vi "SPD.Strobe Phase setup.vi"(5 "Graph":refnum<vi>, 7 "Progress":refnum<vi>, 8 "Error In":errorcluster, 11 "SPD.Stand Ctrl in":T1 {"spdDeviceSession"."hidSPD.Controller"."HV_bias" format="%#_6p, V"; "spdDeviceSession"."hidSPD.Controller"."TSet" format="%#_6p, DegC"}) -> (0 "Error Out":errorcluster, 1 "pass":bool, 2 "result":string, 3 "SPD.Stand Ctrl out":T1 {"spdDeviceSession"."hidSPD.Controller"."HV_bias" format="%#_6p, V"; "spdDeviceSession"."hidSPD.Controller"."TSet" format="%#_6p, DegC"})   [LabVIEW 2018]
uses:
  typedefs/SPD.Stand Ctrl.ctl
  Instruments/SPD HID Interface/hidSPDLibForLabView/LibVIs/hidSPD Controls/hidSPD Device Session.ctl
  Instruments/SPD HID Interface/hidSPDLibForLabView/LibVIs/hidSPD Controls/hidSPD Controller.ctl
  Instruments/KC705 DevBoard/typedefs/DevB.Session.ctl
  Instruments/KeySight 53230A/typedefs/FreqC.Session.ctl
  Instruments/KeySight 8164B/KeySight 8164B LAN InstrLib/typedefs/KeySight 8164B control.ctl
  Instruments/LeCroy SDA830/typedefs/LeCroy.Session.ctl
  typedefs/SPD.Events.ctl
  Instruments/KeySight 8164B/KeySight 8164B LAN InstrLib/typedefs/KeySight 8164B Power Unit.ctl
  <vilib>/Utility/error.llb/Error Cluster From Error Code.vi
  <vilib>/ErrorRing/Error Ring.xnode
  Instruments/KeySight 8164B/KeySight 8164B LAN InstrLib.lvlib
  Instruments/SPD HID Interface/hidSPDLibForLabView/hidSPDLibForLabView.lvlib
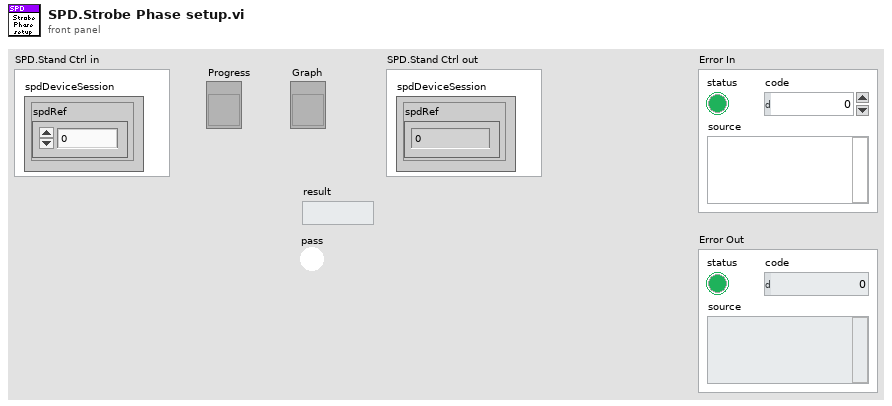
[diagram p1: front panel]
types:
  T1 = typedef "SPD.Stand Ctrl.ctl" = cluster{"spdDeviceSession":T2, "DevBSession":T4, "FreqCSession":T5, "8164BSession":T6, "LeCroySession":T7, "Events":T8}
  T2 = typedef "hidSPDLibForLabView.lvlib/hidSPD Device Session.ctl" = cluster{"spdRef":u64, "connected":bool, "spdName":string, "hidSPD.Controller":T3}
  T3 = typedef "hidSPDLibForLabView.lvlib/hidSPD Controller.ctl" = cluster{"TSet":sgl, "HV_bias":sgl, "DDS_stb_code":u16}
  T4 = typedef "DevB.Session.ctl" = cluster{"DevBRef":refnum<visa-resource-name>, "connected":bool}
  T5 = typedef "FreqC.Session.ctl" = cluster{"FreqCRef":refnum<visa-resource-name>, "timeout":dbl, "connected":bool}
  T6 = typedef "KeySight 8164B LAN InstrLib.lvlib/KeySight 8164B control.ctl" = cluster{"Connection ID":refnum<k5>, "Connected":bool, "Info":string, "Slots Info":string[]}
  T7 = typedef "LeCroy.Session.ctl" = cluster{"LeCroySession":refnum<visa-resource-name>, "connected":bool}
  T8 = typedef "SPD.Events.ctl" = cluster{"DCRTest":refnum<user-event>, "Stop":refnum<user-event>}
  T9 = typedef "KeySight 8164B LAN InstrLib.lvlib/KeySight 8164B Power Unit.ctl" = enum16{"dBm", "Watt"}
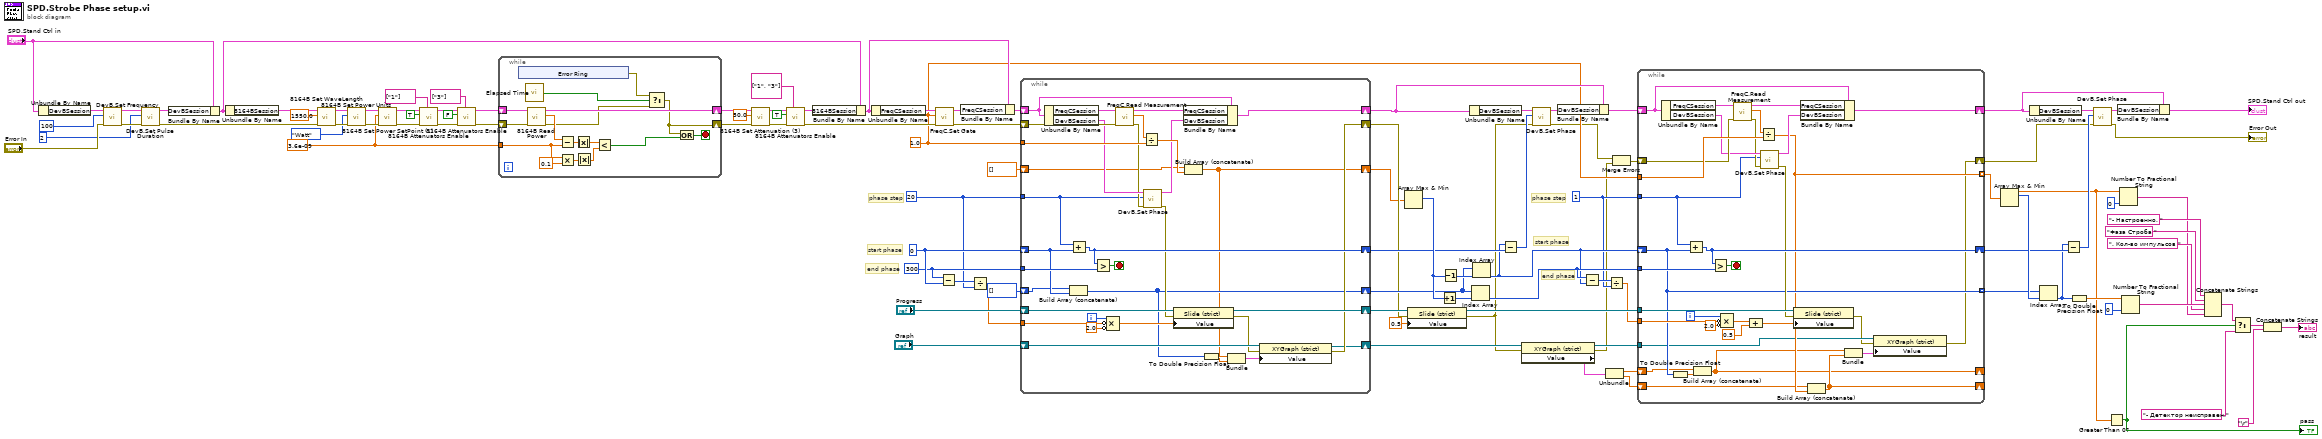
[diagram p0: block diagram]
diagram:
  w15 = 1 ("delta")
  w77 = 3.6e-09 ("Power")
  w45 = 1.0 ("Gate, sec")
  w25 = 20 ("delta")
  w27 = 300 ("HV_bias")
  w28 = 0 ("HV_bias")
  # "end phase"
  # "start phase"
  # "phase step"
  # "end phase"
  # "start phase"
  # "phase step"
  n1 = Unbundle By Name("SPD.Stand Ctrl in") -> ("DevBSession"=w94:T4)
  n2 = call "DevB.Set Frequency.vi"("error in (no error)"="Error In", "Frequency"=100, "DevB Session in"=w94) -> ("error out"=w90:errorcluster, "DevB Session out"=w91:T4)  [unwired: 7 in]
  n3 = call "DevB.Set Pulse Duration.vi"("error in (no error)"=w90, "Pulse Duration"=2, "DevB Session in"=w91) -> ("error out"=w78:errorcluster, "DevB Session out"=w69:T4)  [unwired: 7 in]
  n4 = Bundle By Name(cluster="SPD.Stand Ctrl in", "DevBSession"=w69) -> (w68:T1)
  n5 = Unbundle By Name(w68) -> ("8164BSession"=w67:T6)
  n6 = call "8164B Set WaveLength.vi"("error in"=w78, "WaveLength, nm"=1550.0, "KeySight 8164B control in"=w67) -> ("error out"=w86:errorcluster, "KeySight 8164B control out"=w87:T6)  [unwired: 7 in]
  n7 = call "8164B Set Power Units.vi"("error in"=w86, "Power Unit"=KeySight_8164B_Power_Unit."Watt", "KeySight 8164B control in"=w87) -> ("error out"=w84:errorcluster, "KeySight 8164B control out"=w85:T6)  [unwired: 7 in]
  n8 = call "8164B Set Power SetPoint (1).vi"("error in"=w84, "Power Set Point"=w77, "KeySight 8164B control in"=w85) -> ("error out"=w82:errorcluster, "KeySight 8164B control out"=w83:T6)  [unwired: 7 in]
  n9 = call "8164B Attenuators Enable.vi"("Slots"=string[] ["1"], "error in"=w82, "Enable"=TRUE, "KeySight 8164B control in"=w83) -> ("error out"=w58:errorcluster, "KeySight 8164B control out"=w60:T6)  [unwired: 6 in]
  n10 = call "8164B Attenuators Enable.vi"("Slots"=string[] ["3"], "error in"=w58, "Enable"=FALSE, "KeySight 8164B control in"=w60) -> ("error out"=w57:errorcluster, "KeySight 8164B control out"=w59:T6)  [unwired: 6 in]
  n11 = while {
    shift-right: [w122] -> w75
    shift-left: w59 -> [w124]
    shift-right: [w111] -> w74
    shift-left: w57 -> [w123]
    tunnel: w77 -> [w115]
    stop <- w113 stop-if-true
    n12 = xnode "Error Ring"() -> ("error out"=w109:errorcluster)
    n13 = call "Elapsed Time"() -> ("Time has Elapsed"=w110:bool)  [unwired: 12 in, 7 out]
    n14 = call "8164B Read Power.vi"("error in"=w123, "KeySight 8164B control in"=w124) -> ("error out"=w112:errorcluster, "Power"=w116:dbl, "KeySight 8164B control out"=w122:T6)  [unwired: 7 in]
    n15 = Subtract(x=w116, y=w115) -> (x-y=w121:dbl)
    n16 = Multiply(x=w115, y=0.1) -> (x*y=w119:dbl)
    n17 = Absolute Value(x=w121) -> (abs(x)=w118:dbl)
    n18 = Absolute Value(x=w119) -> (abs(x)=w117:dbl)
    n19 = Less?(x=w118, y=w117) -> (x < y?=w114:bool)
    n20 = Select(t=w109, s=w110, f=w112) -> (s? t:f=w111:errorcluster)
    n21 = Compound Arithmetic op=OR(w111, w114) -> (w113:bool)
  }
  n22 = call "8164B Set Attenuation (3).vi"("error in"=w74, "Att 3, dB"=50.0, "KeySight 8164B control in"=w75) -> ("error out"=w72:errorcluster, "KeySight 8164B control out"=w73:T6)  [unwired: 7 in]
  n23 = call "8164B Attenuators Enable.vi"("Slots"=string[] ["1", "3"], "error in"=w72, "Enable"=TRUE, "KeySight 8164B control in"=w73) -> ("error out"=w64:errorcluster, "KeySight 8164B control out"=w66:T6)  [unwired: 6 in]
  n24 = Bundle By Name(cluster=w68, "8164BSession"=w66) -> (w63:T1)
  n25 = Unbundle By Name(w63) -> ("FreqCSession"=w65:T5)
  n26 = call "FreqC.Set Gate.vi"("error In"=w64, "Gate, sec"=w45, "FreqC Session in"=w65) -> ("error out"=w102:errorcluster, "FreqC Session out"=w62:T5)  [unwired: 7 in]
  n27 = Subtract(x=w27, y=w28) -> (x-y=w26:i32)
  n28 = Bundle By Name(cluster=w63, "FreqCSession"=w62) -> (w61:T1)
  n29 = Divide(x=w26, y=w25) -> (x/y=w23:dbl)
  n30 = while {
    shift-right: [w136] -> w21
    shift-left: w102 -> [w157]
    shift-right: [w162] -> w48
    shift-left: w61 -> [w156]
    tunnel: w45 -> [w159]
    tunnel: w25 -> [w147]
    shift-right: [w149] -> w51
    shift-left: w28 -> [w148]
    tunnel: w27 -> [w151]
    shift-right: [w144] -> w22
    shift-left: "Progress" -> [w146]
    tunnel: w23 -> [w142]
    shift-right: [w130] -> w8
    shift-left: dbl[] [] -> [w139]
    shift-right: [w135] -> w10
    shift-left: "Graph" -> [w138]
    shift-right: [w131] -> w35
    shift-left: i32[] [] ("HV_bias") -> [w133]
    i -> [w143]
    stop <- w150 stop-if-true
    n31 = Unbundle By Name(w156) -> ("FreqCSession"=w161:T5, "DevBSession"=w153:T4)
    n32 = Build Array (concatenate)(w133, w148) -> (w131:i32[])
    n33 = Add(x=w147, y=w148) -> (x+y=w149:i32)
    n34 = Greater?(x=w149, y=w151) -> (0:w150:bool)
    n35 = Compound Arithmetic op=MULTIPLY(w143, invert w142, invert 2.0 ("value")) -> (w140:dbl)
    n36 = call "FreqC.Read Measurement.vi"("error In"=w157, "FreqC Session in"=w161) -> ("error out"=w152:errorcluster, "Measurement"=w160:dbl, "FreqC Session out"=w155:T5)  [unwired: 7 in]
    n37 = Divide(x=w160, y=w159) -> (x/y=w158:dbl)
    n38 = call "DevB.Set Phase.vi"("error in (no error)"=w152, "Phase"=w147, "DevB Session in"=w153) -> ("error out"=w145:errorcluster, "DevB Session out"=w154:T4)  [unwired: 7 in]
    n39 = property class="Slide (strict)"(reference=w146, error in=w145, "Value"=w140) -> (reference out=w144:refnum<vi>, error out=w137:errorcluster)
    n40 = Bundle By Name(cluster=w156, "FreqCSession"=w155, "DevBSession"=w154) -> (w162:T1)
    n41 = Build Array (concatenate)(w139, w158) -> (w130:dbl[])
    n42 = To Double Precision Float(number=w131) -> (double precision float=w132:dbl[])
    n43 = Bundle(w132, w130) -> (w134:cluster{dbl[], dbl[]})  [unwired: 1 in]
    n44 = property class="XYGraph (strict)"(reference=w138, error in=w137, "Value"=w134) -> (reference out=w135:refnum<vi>, error out=w136:errorcluster)
  }
  n45 = Array Max & Min(array=w8) -> (max index (indices)=w52:i32)  [unwired: 3 out]
  n46 = property class="Slide (strict)"(reference=w22, error in=w21, "Value"=0.5) -> (reference out=w19:refnum<vi>, error out=w9:errorcluster)
  n47 = Increment(x=w52) -> (x+1=w54:i32)
  n48 = Decrement(x=w52) -> (x-1=w53:i32)
  n49 = Unbundle By Name(w48) -> ("DevBSession"=w50:T4)
  n50 = Index Array(array=w35, index=w54) -> (element=w18:i32)
  n51 = Index Array(array=w35, index=w53) -> (element=w17:i32)
  n52 = Subtract(x=w17, y=w51) -> (x-y=w47:i32)
  n53 = property class="XYGraph (strict)"(reference=w10, error in=w9) -> (reference out=w3:refnum<vi>, error out=w1:errorcluster, "Value"=w6:cluster{dbl[], dbl[]})
  n54 = call "DevB.Set Phase.vi"("error in (no error)"=w9, "Phase"=w47, "DevB Session in"=w50) -> ("error out"=w44:errorcluster, "DevB Session out"=w49:T4)  [unwired: 7 in]
  n55 = Bundle By Name(cluster=w48, "DevBSession"=w49) -> (w46:T1)
  n56 = Subtract(x=w18, y=w17) -> (x-y=w16:i32)
  n57 = Unbundle(w6) -> (w5:dbl[], w4:dbl[])
  n58 = Divide(x=w16, y=w15) -> (x/y=w14:dbl)
  n59 = Merge Errors(w44, w1) -> (w2:errorcluster)
  n60 = while {
    shift-right: [w167] -> w37
    shift-left: w2 -> [w191]
    shift-right: [w195] -> w39
    shift-left: w46 -> [w190]
    tunnel: w45 -> [w192]
    tunnel: w15 -> [w163]
    shift-right: [w183] -> w42
    shift-left: w17 -> [w173]
    tunnel: w18 -> [w185]
    tunnel: [w173] -> w34 mode=indexing
    tunnel: w19 -> [w182]
    tunnel: w14 -> [w179]
    tunnel: [w171] -> w7 mode=indexing
    shift-right: [w164] -> _
    shift-left: w5 -> [w172]
    shift-right: [w166] -> _
    shift-left: w4 -> [w170]
    tunnel: w3 -> [w169]
    i -> [w180]
    stop <- w184 stop-if-true
    n61 = Unbundle By Name(w190) -> ("FreqCSession"=w194:T5, "DevBSession"=w187:T4)
    n62 = To Double Precision Float(number=w173) -> (double precision float=w174:dbl)
    n63 = Add(x=w163, y=w173) -> (x+y=w183:i32)
    n64 = Build Array (concatenate)(w172, w174) -> (w164:dbl[])
    n65 = Greater?(x=w183, y=w185) -> (0:w184:bool)
    n66 = Compound Arithmetic op=MULTIPLY(w180, invert w179, invert 2.0 ("value")) -> (w177:dbl)
    n67 = call "FreqC.Read Measurement.vi"("error In"=w191, "FreqC Session in"=w194) -> ("error out"=w186:errorcluster, "Measurement"=w193:dbl, "FreqC Session out"=w189:T5)  [unwired: 7 in]
    n68 = Compound Arithmetic op=ADD(w177, 0.5 ("value")) -> (w175:dbl)
    n69 = Divide(x=w193, y=w192) -> (x/y=w171:dbl)
    n70 = call "DevB.Set Phase.vi"("error in (no error)"=w186, "Phase"=w163, "DevB Session in"=w187) -> ("error out"=w181:errorcluster, "DevB Session out"=w188:T4)  [unwired: 7 in]
    n71 = property class="Slide (strict)"(reference=w182, error in=w181, "Value"=w175) -> (error out=w168:errorcluster)  [unwired: 1 out]
    n72 = Bundle By Name(cluster=w190, "FreqCSession"=w189, "DevBSession"=w188) -> (w195:T1)
    n73 = Build Array (concatenate)(w170, w171) -> (w166:dbl[])
    n74 = Bundle(w164, w166) -> (w165:cluster{dbl[], dbl[]})  [unwired: 1 in]
    n75 = property class="XYGraph (strict)"(reference=w169, error in=w168, "Value"=w165) -> (error out=w167:errorcluster)  [unwired: 1 out]
  }
  n76 = Array Max & Min(array=w7) -> (max value=w30:dbl, max index (indices)=w43:i32)  [unwired: 2 out]
  n77 = Unbundle By Name(w39) -> ("DevBSession"=w41:T4)
  n78 = Index Array(array=w34, index=w43) -> (element=w33:i32)
  n79 = Subtract(x=w33, y=w42) -> (x-y=w38:i32)
  n80 = To Double Precision Float(number=w33) -> (double precision float=w32:dbl)
  n81 = call "DevB.Set Phase.vi"("error in (no error)"=w37, "Phase"=w38, "DevB Session in"=w41) -> ("error out"=→"Error Out":errorcluster, "DevB Session out"=w40:T4)  [unwired: 7 in]
  n82 = Greater Than 0?(x=w30) -> (x > 0?=w29:bool)
  "pass" <- w29
  n83 = Bundle By Name(cluster=w39, "DevBSession"=w40) -> (→"SPD.Stand Ctrl out":T1)
  n84 = Number To Fractional String(number=w30, precision (6)=i16 0) -> (F-format string=w95:string)  [unwired: 2 in]
  n85 = Number To Fractional String(number=w32, precision (6)=i16 0) -> (F-format string=w98:string)  [unwired: 2 in]
  n86 = Concatenate Strings("- Настроенно. " ("report"), "Фаза Строба " ("report"), w98, ". Кол-во импульсов " ("report"), w95) -> (w101:string)
  n87 = Select(t=w101, s=w29, f="- Детектор неисправен.") -> (s? t:f=w106:string)
  n88 = Concatenate Strings(w106, "\r") -> (→"result":string)
